vi "Hardware in the Loop - Start Shot.vi"(8 "error in":errorcluster, 11 "Address":string) -> (0 "error out":errorcluster, 2 "Shot Completed":bool)   [LabVIEW 2017, in "Communications Library.lvlib"]
doc: "Start a shot, by connecting to the appropriate port number and waiting until the \"Shot_Complete\" message is received."
uses:
  Communications Library.lvlib
  Typedefs/Functional Global Variable Action--Enum.ctl
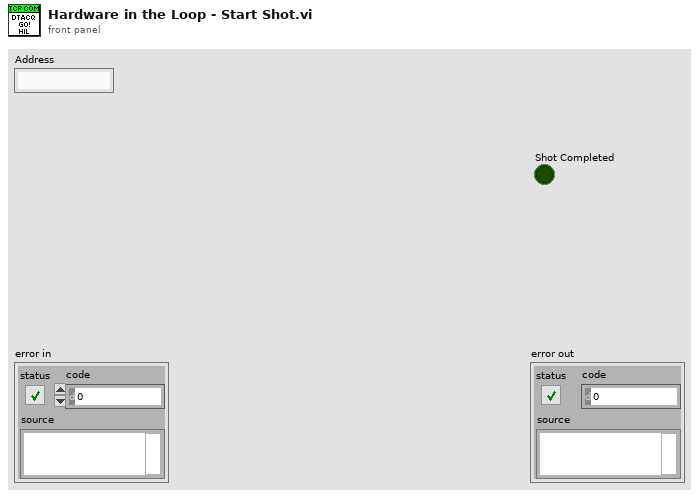
[diagram p1: front panel]
types:
  T1 = typedef "Communications Library.lvlib/Functional Global Variable Action--Enum.ctl" = enum16{"Initialise", "Write Module Config", "Write Carrier Config", "Read"}
  T2 = typedef "Communications Library.lvlib/DTACQ Module Carrier Configuration--Cluster.ctl" = cluster{"Name":string, "IP":string, "Control Port":i32, "Timeout (ms)":i32, "Continuous Capture Port (Multiplexed)":i32, "Start HIL Shot Port":i32, "AWG Upload Port (Multiplexed)":i32, "Download Captured Data Port (Multiplexed)":i32, "Module Slots":i32, "Module Configurations":T3[]}
  T3 = typedef "Communications Library.lvlib/DTACQ Module Configuration--Cluster.ctl" = cluster{"Name":string, "Position":string, "Module Type":T4, "Control Port":i32, "Timeout (ms)":i32, "Channels":i32}
  T4 = typedef "Communications Library.lvlib/DTACQ Device Type--Enum.ctl" = enum16{"Carrier", "Analog In Module", "Analog Out Module", "Generic Module"}
  T5 = typedef "Communications Library.lvlib/DTACQ Connection Data--Cluster.ctl" = cluster{"Description":string, "Address":string, "Port":u16, "timeout (ms)":i32, "Termination Character":string, "TCP Connection Reference":refnum<k5>, "Open Connection":bool}
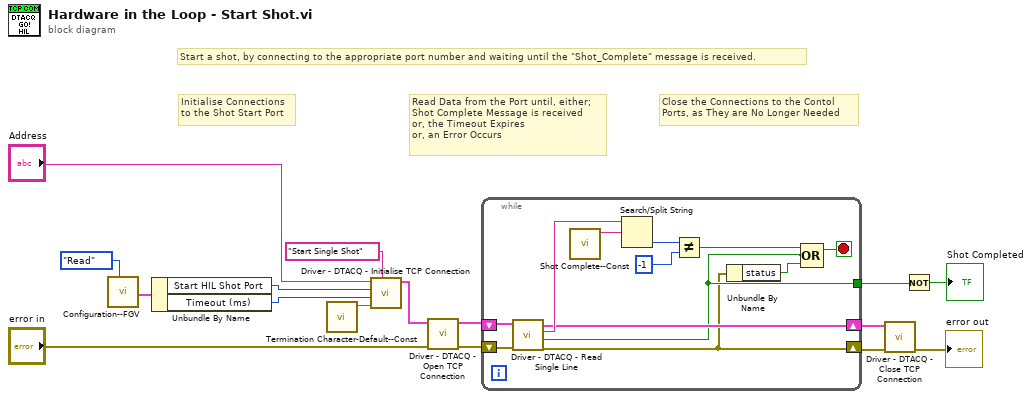
[diagram p0: block diagram]
diagram:
  # "Start a shot, by connecting to the appropriate port number and waiting until the \"Shot_Complete\" message is received."
  # "Close the Connections to the Contol\nPorts, as They are No Longer Needed"
  # "Read Data from the Port until, either;\nShot Complete Message is received\nor, the Timeout Expires\nor, an Error Occurs"
  # "Initialise Connections\nto the Shot Start Port"
  n1 = call "Configuration--FGV.vi"("Functional Global Action"=Functional_Global_Variable_Action--Enum."Read") -> ("Carrier Configuration Out"=w3:T2)  [unwired: 9 in, 1 out]
  n2 = Unbundle By Name(w3) -> ("Start HIL Shot Port"=w2:i32, "Timeout (ms)"=w1:i32)
  n3 = call "Termination Character-Default--Const.vi"() -> ("Termination Character"=w7:string)  [unwired: 11 in]
  n4 = call "Driver - DTACQ - Initialise TCP Connection.vi"("Description"="Start Single Shot", "Termination Character"=w7, "timeout (ms)"=w1, "Port"=w2, "Address"="Address") -> ("DTACQ Connection Data Out"=w15:T5)  [unwired: 6 in]
  n5 = call "Driver - DTACQ - Open TCP Connection.vi"("error in"="error in", "DTACQ Connection Data In"=w15) -> ("error out"=w6:errorcluster, "DTACQ Connection Data Out"=w5:T5)  [unwired: 8 in]
  n6 = while {
    shift-right: [w23] -> w14
    shift-left: w5 -> [w22]
    shift-right: [w18] -> w12
    shift-left: w6 -> [w28]
    tunnel: [w20] -> w10
    stop <- w19 stop-if-true
    n7 = call "Driver - DTACQ - Read Single Line.vi"("error in"=w28, "DTACQ Connection Data In"=w22) -> ("error out"=w18:errorcluster, "Timed Out"=w20:bool, "Read String"=w27:string, "DTACQ Connection Data Out"=w23:T5)  [unwired: 6 in]
    n8 = call "Shot Complete--Const.vi"() -> ("Shot Complete Message"=w26:string)  [unwired: 11 in]
    n9 = Search/Split String(string=w27, search string/char (-)=w26) -> (offset of match=w25:i32)  [unwired: 1 in, 2 out]
    n10 = Not Equal?(x=w25, y=-1) -> (x != y?=w21:bool)
    n11 = Unbundle By Name(w18) -> ("status"=w17:bool)
    n12 = Compound Arithmetic op=OR(w21, w20, w17) -> (w19:bool)
  }
  n13 = call "Driver - DTACQ - Close TCP Connection.vi"("error in"=w12, "DTACQ Connection Data In"=w14) -> ("error out"=→"error out":errorcluster)  [unwired: 8 in, 1 out]
  n14 = Not(x=w10) -> (.not. x?=→"Shot Completed":bool)
